vi "LocalizeVI.vi"(8 "error in (no error)":errorcluster, 9 "Target Language":string, 10 "Dictionary":T1, 11 "VI in":refnum<vi>) -> (0 "error out":errorcluster)   [LabVIEW 2019]
uses:
  Dictionary--Cluster.ctl
  Font -- Cluster.ctl
  Phrase Dictionary Entry -- Cluster.ctl
  <vilib>/Utility/traverseref.llb/TRef TravTarget.ctl
  <vilib>/Utility/traverseref.llb/VI Scripting - Traverse.lvlib
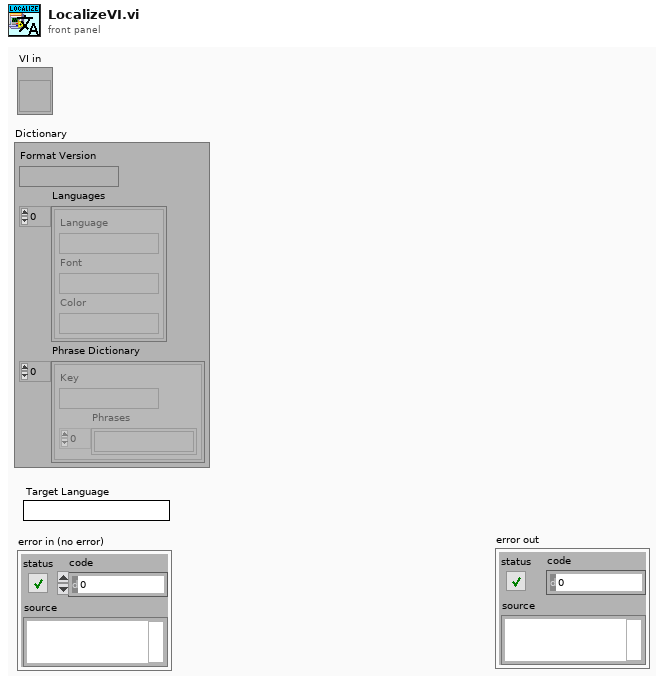
[diagram p1: front panel]
types:
  T1 = typedef "Dictionary--Cluster.ctl" = cluster{"Format Version":string, "Languages":T2[], "Phrase Dictionary":T3[]}
  T2 = typedef "Font -- Cluster.ctl" = cluster{"Language":string, "Font":string, "Color":string}
  T3 = typedef "Phrase Dictionary Entry -- Cluster.ctl" = cluster{"Key":string, "Phrases":string[]}
  T4 = typedef "TRef TravTarget.ctl" = enum16{"FP", "BD", "Other"}
  T5 = typedef "Font Info -- Cluster.ctl" = cluster{"Custom Font Color":bool, "Font Color":u32, "Custom Font Name":bool, "Font Name":string}
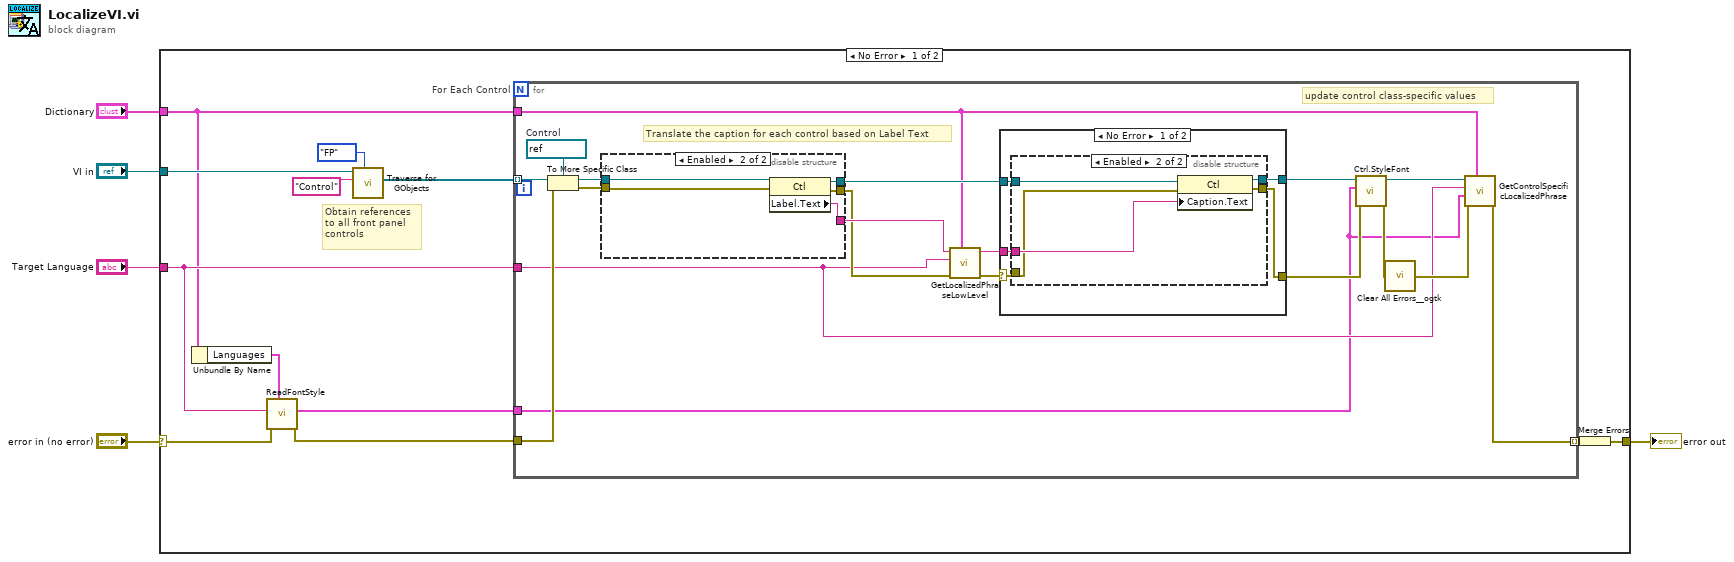
[diagram p0: block diagram]
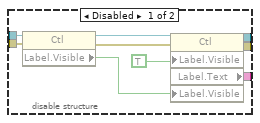
[diagram p2: hidden frame]
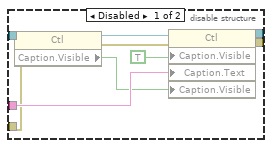
[diagram p3: hidden frame]
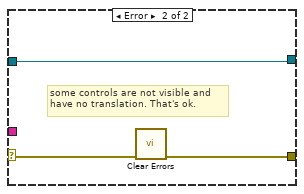
[diagram p4: hidden frame]
diagram:
  n1 = case shown="No Error" "error in (no error)" {
    selector: "error in (no error)" -> [w9 w73]
    tunnel: "VI in" -> [w15 _]
    tunnel: [w12 w73] -> w4
    tunnel: "Dictionary" -> [w7 _]
    tunnel: "Target Language" -> [w10 _]
    frame No Error {
      # "Obtain references to all front panel controls"
      n2 = Unbundle By Name(w7) -> ("Languages"=w6:T2[])
      n3 = call "ReadFontStyle.vi"("Fonts"=w6, "error in (no error)"=w9, "Target Language"=w10) -> ("error out"=w11:errorcluster, "Font Info"=w8:T5)  [unwired: 7 in]
      n4 = call <vilib>:"Traverse for GObjects.vi"("Traverse Target"=TRef_TravTarget."FP", "Class Name"="Control", "VI Refnum"=w15) -> ("References"=w16:refnum<vi>[])  [unwired: 5 in, 3 out]
      n5 = for "For Each Control" {
        tunnel: w16 -> [w36] mode=indexing
        tunnel: w11 -> [w34]
        tunnel: w7 -> [w26]
        tunnel: w10 -> [w23]
        tunnel: [w25] -> w17 mode=indexing
        tunnel: w8 -> [w18]
        w35 = refnum<vi> refnum  # Control
        # "update control class-specific values"
        # "Translate the caption for each control based on Label Text"
        n6 = To More Specific Class(target class=w35, reference=w36, error in=w34) -> (specific class reference=w32:refnum<vi>, error out=w29:errorcluster)
        n7 = disable-structure shown="Enabled" {
          disable-tunnel: [w45 w50] -> w33
          disable-tunnel: w32 -> [w44 w46]
          disable-tunnel: [w40 w49] -> w30
          disable-tunnel: w29 -> [w39 w47]
          disable-tunnel: [w37 w48] -> w28
          frame Disabled {
            n8 = property class="Ctl"(reference=w44, error in=w39) -> (reference out=w43:refnum<vi>, error out=w38:errorcluster, "Label.Visible"=w42:bool)
            n9 = property class="Ctl"(reference=w43, error in=w38, "Label.Visible"=TRUE, "Label.Visible"=w42) -> (reference out=w40:refnum<vi>, error out=w37:errorcluster, "Label.Text"=w45:string)
          }
          frame Enabled {
            n10 = property class="Ctl"(reference=w46, error in=w47) -> (reference out=w49:refnum<vi>, error out=w48:errorcluster, "Label.Text"=w50:string)
          }
        }
        n11 = call "GetLocalizedPhraseLowLevel.vi"("Dictionary"=w26, "error in (no error)"=w28, "Target Language"=w23, "Key"=w33) -> ("error out"=w27:errorcluster, "Localized Phrase"=w31:string)  [unwired: 6 in]
        n12 = case shown="No Error" w27 {
          selector: w27 -> [w52 w72]
          tunnel: w31 -> [w55 _]
          tunnel: w30 -> [w54 w70]
          tunnel: [w53 w71] -> w20
          tunnel: [w51 w70] -> w22
          frame No Error {
            n13 = disable-structure shown="Enabled" {
              disable-tunnel: w55 -> [w63 w69]
              disable-tunnel: w54 -> [w62 w66]
              disable-tunnel: [w58 w68] -> w53
              disable-tunnel: w52 -> [w57 w65]
              disable-tunnel: [w56 w67] -> w51
              frame Disabled {
                n14 = property class="Ctl"(reference=w62, error in=w57) -> (reference out=w61:refnum<vi>, error out=w59:errorcluster, "Caption.Visible"=w60:bool)
                n15 = property class="Ctl"(reference=w61, error in=w59, "Caption.Visible"=TRUE, "Caption.Text"=w63, "Caption.Visible"=w60) -> (reference out=w56:refnum<vi>, error out=w58:errorcluster)
              }
              frame Enabled {
                n16 = property class="Ctl"(reference=w66, error in=w65, "Caption.Text"=w69) -> (reference out=w67:refnum<vi>, error out=w68:errorcluster)
              }
            }
          }
          frame Error {
            # "some controls are not visible and \nhave no translation. That's ok."
            n17 = call <vilib>:"Clear Errors.vi"("error in (no error)"=w72) -> ("error out"=w71:errorcluster)  [unwired: 5 in, 1 out]
          }
        }
        n18 = call "Ctrl.StyleFont.vi"("error in (no error)"=w20, "Font Info"=w18, "Ctl Ref in"=w22) -> ("error out"=w19:errorcluster, "Ctl Ref out"=w21:refnum<vi>)  [unwired: 7 in]
        n19 = call <userlib>:"Clear All Errors__ogtk.vi"("Error In"=w19) -> ("Error Out"=w24:errorcluster)  [unwired: 3 in]
        n20 = call "GetControlSpecificLocalizedPhrase.vi"("Dictionary"=w26, "error in (no error)"=w24, "Font Info"=w18, "Target Language"=w23, "Control Reference"=w21) -> ("error out"=w25:errorcluster)  [unwired: 5 in, 1 out]
      }
      n21 = Merge Errors(w17) -> (w12:errorcluster)
    }
    frame Error {
    }
  }
  "error out" <- w4
